vi "Start LogData.vi"(8 "error in":errorcluster, 9 "LogData":bool, 10 "File Path":path, 11 "Data in":T1 {"LogStartTime" format="%<%x %.3X>T"}) -> (0 "error out":errorcluster, 3 "Data Out":T1 {"LogStartTime" format="%<%x %.3X>T"})   [LabVIEW 2023]
uses:
  controls/UI Data.ctl
  <vilib>/NI/Modbus Library/API/Master/Modbus Master.lvclass
  LibreVNA/LibreVNA.lvclass
  <vilib>/Utility/file.llb/Write Delimited Spreadsheet (string).vi
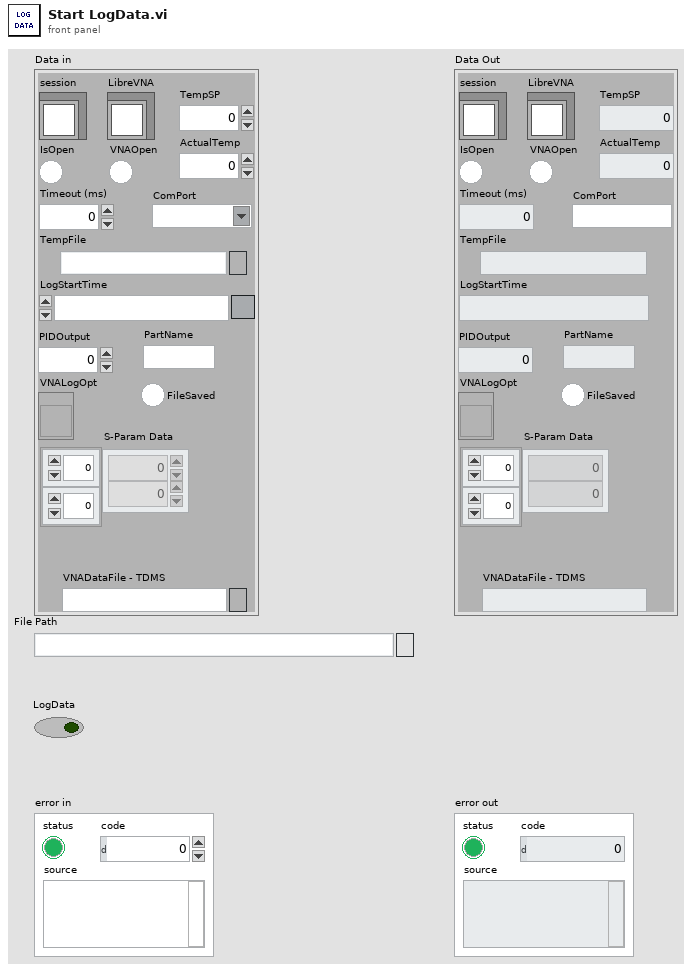
[diagram p1: front panel]
types:
  T1 = typedef "UI Data.ctl" = cluster{"session":refnum<class "Modbus Master.lvclass">, "IsOpen":bool, "Timeout (ms)":i32, "TempFile":path, "LogStartTime":timestamp, "LibreVNA":refnum<class "LibreVNA.lvclass">, "VNAOpen":bool, "TempSP":dbl, "ActualTemp":dbl, "FileSaved":bool, "PIDOutput":dbl, "VNALogOpt":refnum<vi>, "PartName":string, "ComPort":refnum<visa-resource-name>, "S-Param Data":dbl[][], "VNADataFile - TDMS":path}
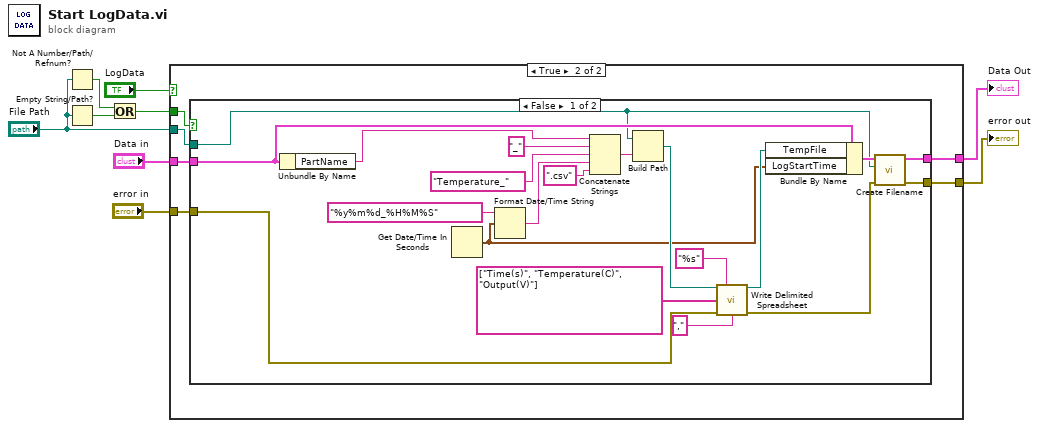
[diagram p0: block diagram]
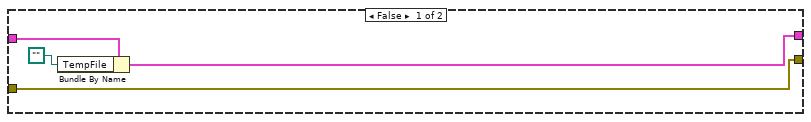
[diagram p2: hidden frame]
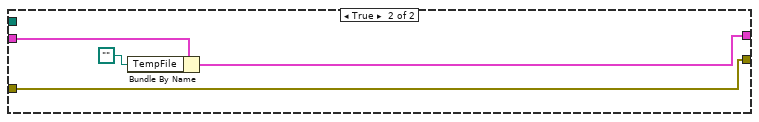
[diagram p3: hidden frame]
diagram:
  n1 = Not A Number/Path/Refnum?(number/path/refnum="File Path") -> (NaN/Path/Refnum?=w4:bool)
  n2 = Empty String/Path?(string/path="File Path") -> (empty?=w3:bool)
  n3 = Or(x=w4, y=w3) -> (x .or. y?=w2:bool)
  n4 = case shown="True" "LogData" {
    tunnel: "File Path" -> [_ w19]
    tunnel: [w12 w17] -> w8
    tunnel: "Data in" -> [w13 w18]
    tunnel: "error in" -> [w10 w16]
    tunnel: [w10 w15] -> w1
    tunnel: w2 -> [_ w14]
    frame False {
      n5 = Bundle By Name(cluster=w13, "TempFile"=path "") -> (w12:T1)
    }
    frame True {
      n6 = case shown="False" w14 {
        tunnel: w19 -> [w22 _]
        tunnel: w18 -> [w27 w42]
        tunnel: [w21 w41] -> w17
        tunnel: w16 -> [w29 w43]
        tunnel: [w20 w43] -> w15
        frame False {
          n7 = Unbundle By Name(w27) -> ("PartName"=w26:string)
          n8 = Get Date/Time In Seconds() -> (seconds since 1Jan1904=w28:timestamp)
          n9 = Format Date/Time String(time format string (%c)="%y%m%d_%H%M%S", seconds (now)=w28) -> (date/time string=w38:string)  [unwired: 1 in]
          n10 = Concatenate Strings(w26, "_" ("string"), "Temperature_" ("string"), w38, ".csv" ("string")) -> (w35:string)
          n11 = Build Path(base path=w22, name or relative path=w35) -> (appended path=w34:path)
          n12 = call-poly <vilib>:"Write Delimited Spreadsheet.vi"("file path (dialog if empty)"=w34, "format (%s)"="%s", "1D data"=string[] ["Time(s)", "Temperature(C)", "Output(V)"], "error in (no error)"=w29, "delimiter (\\t)"="," ("delimiter (\\t)")) -> ("new file path (Not A Path if cancelled)"=w33:path, "error out"=w23:errorcluster)  [unwired: 9 in]
          n13 = Bundle By Name(cluster=w27, "TempFile"=w33, "LogStartTime"=w28) -> (w24:T1)
          n14 = call "Create Filename.vi"("error in"=w23, "Path in"=w22, "Data in"=w24) -> ("error out"=w20:errorcluster, "Data Out"=w21:T1)  [unwired: 6 in, 1 out]
        }
        frame True {
          n15 = Bundle By Name(cluster=w42, "TempFile"=path "") -> (w41:T1)
        }
      }
    }
  }
  "Data Out" <- w8
  "error out" <- w1
